vi "SeimensS7Net_Destroy.vi"(8 "error in (no error)":errorcluster caption="错误输入（无错误）", 11 "Seimens 输入":refnum<class "Seimens.lvclass">) -> (0 "error out":errorcluster caption="错误输出")   [LabVIEW 2018, in "Seimens.lvclass"]
uses:
  Seimens.lvclass
  Seimens.lvclass/Seimens.ctl
  D:/LiMing/Labview/lib/LM_HslCommunication/DLL/HslCommunication.dll
  DLL/HslCommunication.dll
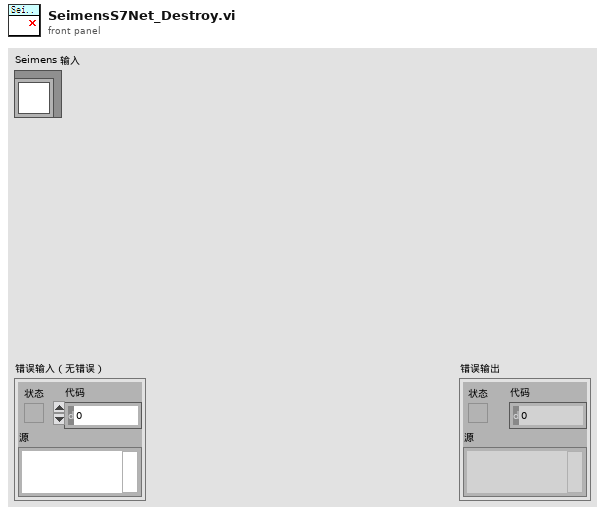
[diagram p1: front panel]
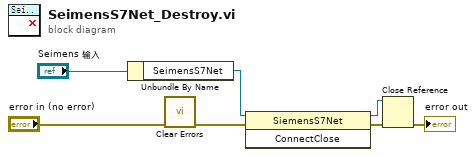
[diagram p0: block diagram]
diagram:
  n1 = Unbundle By Name("Seimens 输入") -> ("SeimensS7Net"=w1:refnum<k24>)
  n2 = call <vilib>:"Clear Errors.vi"("error in (no error)"="error in (no error)") -> ("error out"=w4:errorcluster)  [unwired: 5 in, 1 out]
  n3 = invoke class="SiemensS7Net" method="ConnectClose"(reference=w1, error in=w4) -> (reference out=w6:refnum<k24>, error out=w7:errorcluster)  [unwired: 1 in, 1 out]
  n4 = Close Reference(reference=w6, error in (no error)=w7) -> (error out=→"error out":errorcluster)
